vi "Update Setting.vi"(0 "Bobcat 640 in":refnum<class "Bobcat 640.lvclass">, 1 "Setting":T1, 2 "Value":string, 3 "error in":errorcluster) -> (7 "Bobcat 640 out":refnum<class "Bobcat 640.lvclass">, 8 "Supported?":bool, 10 "error out":errorcluster)   [LabVIEW 2018, in "Bobcat 640.lvlib" / "Bobcat 640.lvclass"]
uses:
  Bobcat 640.lvclass
  PPLs/Camera/Parent/Camera.lvlibp/Custom Controls/Camera Setting.ctl
  PPLs/Camera/Parent/Camera.lvlibp/Camera.lvclass
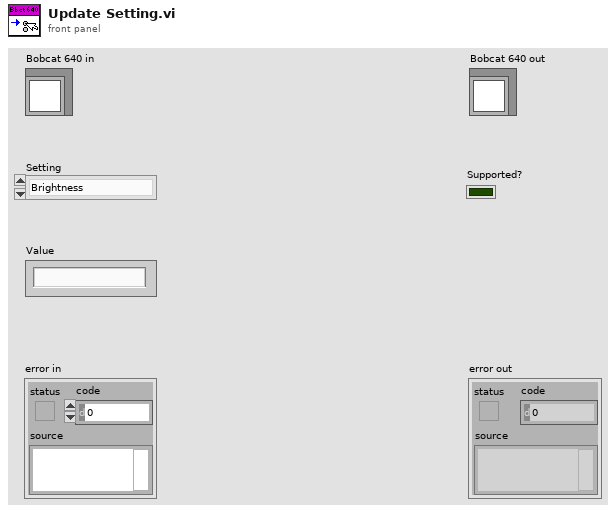
[diagram p1: front panel]
types:
  T1 = typedef "Camera.lvlibp/Camera.lvclass/Camera Setting.ctl" = enum16{"Brightness", "Rotation", "Contrast", "Exposure", "Frame Rate", "Gain", "Gamma", "Image Resolution", "Sharpness"}
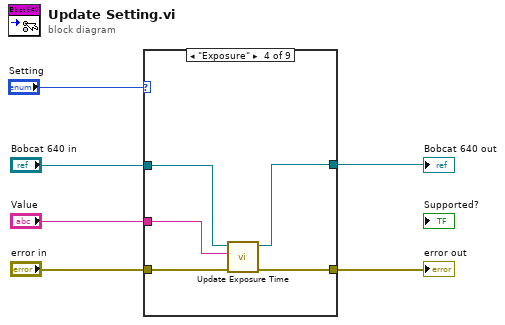
[diagram p0: block diagram]
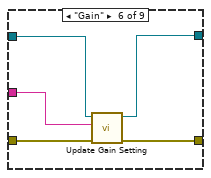
[diagram p6: hidden frame]
diagram:
  n1 = case shown="\"Exposure\"" "Setting" {
    tunnel: "Bobcat 640 in" -> [w7 w10 w12 w17 w19 w22 w26 w28 w30]
    tunnel: [w8 w9 w11 w14 w18 w23 w25 w27 w29] -> w3
    tunnel: "error in" -> [w8 w9 w11 w15 w18 w24 w25 w27 w29]
    tunnel: [w7 w10 w12 w16 w19 w21 w26 w28 w30] -> w2
    tunnel: "Value" -> [_ _ _ w13 _ w20 _ _ _]
    frame "Brightness", Default {
    }
    frame "Rotation" {
    }
    frame "Contrast" {
    }
    frame "Exposure" {
      n2 = call "Update Exposure Time.vi"("error in (no error)"=w15, "Value"=w13, "Bobcat 640 in"=w17) -> ("error out"=w14:errorcluster, "Bobcat 640 out"=w16:refnum<class "Bobcat 640.lvclass">)  [unwired: 7 in]
    }
    frame "Frame Rate" {
    }
    frame "Gain" {
      n3 = call "Update Gain Setting.vi"("error in (no error)"=w24, "Value"=w20, "Bobcat 640 in"=w22) -> ("error out"=w23:errorcluster, "Bobcat 640 out"=w21:refnum<class "Bobcat 640.lvclass">)  [unwired: 7 in]
    }
    frame "Gamma" {
    }
    frame "Image Resolution" {
    }
    frame "Sharpness" {
    }
  }
  "error out" <- w3
  "Bobcat 640 out" <- w2
